vi "SYST_COMM_GPIB_PMET_ADDR.vi"(0 "VISA IN":refnum<visa-resource-name>, 5 "error in":errorcluster, 7 "Address":i32) -> (14 "VISA Out":refnum<visa-resource-name>, 19 "error out":errorcluster)   [LabVIEW 2018, in "PNA-X.lvlib"]
doc: "SYSTem:COMMunicate:GPIB:PMETer:ADDRess <num> \n(Read-Write) Specifies the GPIB address of the power meter to be used in a source power calibration. \nWhen performing a source power cal, the PNA will search VISA interfaces that are configured in the \nAgilent IO LIbraries on the PNA. \nParameters \n<num> GPIB address of the power meter. Choose any integer between 0 and 30. \nExamples SYST:COMM:GPIB:PMET:ADDR 13 \nsystem:communicate:gpib:pmeter:address 14 \nQuery Syntax SYSTem:COMMunicate:GPIB:PMETer:ADDRess? \nReturn Type Numeric \nDefault 13"
uses:
  PNA-X.lvlib
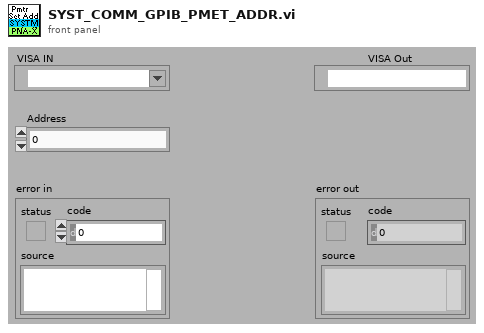
[diagram p1: front panel]
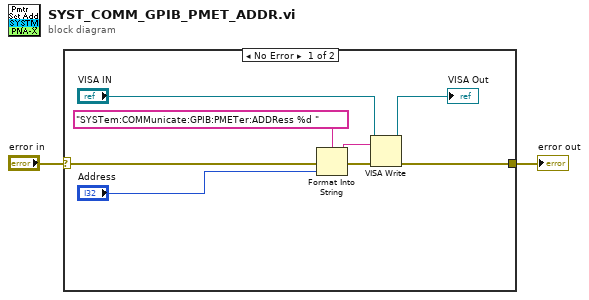
[diagram p0: block diagram]
diagram:
  n1 = case shown="No Error" "error in" {
    selector: "error in" -> [w10 w11]
    tunnel: [w5 w11] -> w1
    frame No Error {
      n2 = Format Into String(format string="SYSTem:COMMunicate:GPIB:PMETer:ADDRess %d " ("Cmdline"), error in=w10, "Address") -> (resulting string=w8:string, error out=w9:errorcluster)  [unwired: 1 in]
      n3 = VISA Write(VISA resource name="VISA IN", write buffer=w8, error in (no error)=w9) -> (VISA resource name out=→"VISA Out":refnum<visa-resource-name>, error out=w5:errorcluster)  [unwired: 1 out]
    }
    frame Error {
    }
  }
  "error out" <- w1
